vi "Modbus PreCondition.vi"(9 "Blower ON/OFF":bool, 10 "Absolute Time":dbl format="%#.20f", 11 "Timing in":T1 {"Absolute Time" format="%<%H:%M:%S%3u>t"; "Display Time" format="%#.20f"; "Test Time Ref" format="%#.20f"; "Precondition Time Ref" format="%#.20f"; "First Call Time Ref" format="%#.20f"}) -> (3 "Timing Out":T1 {"Absolute Time" format="%<%H:%M:%S%3u>t"; "Display Time" format="%#.20f"; "Test Time Ref" format="%#.20f"; "Precondition Time Ref" format="%#.20f"; "First Call Time Ref" format="%#.20f"})   [LabVIEW 2023, in "Modbus.lvlib"]
uses:
  Modbus.lvlib
  Modbus Timing.ctl
  <vilib>/Utility/miscctls.llb/LVDateTimeRec.ctl
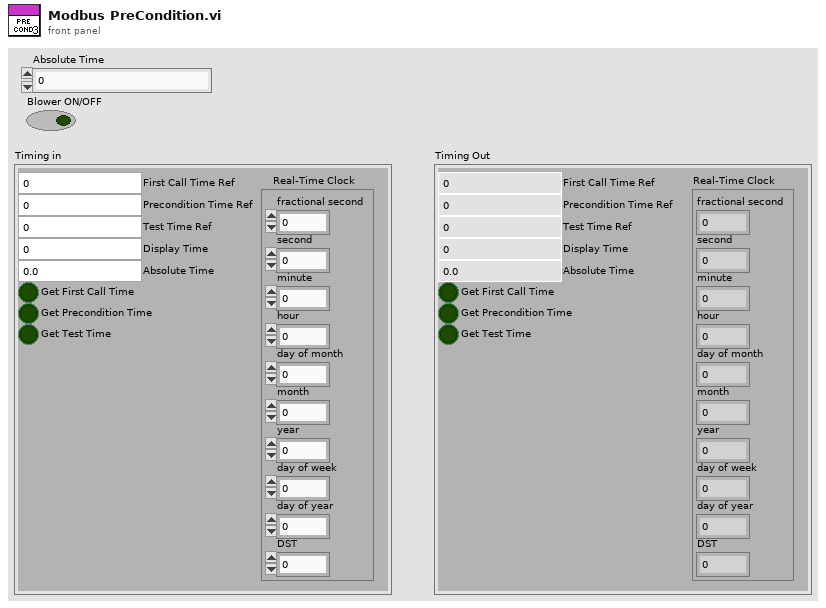
[diagram p1: front panel]
types:
  T1 = typedef "Modbus Timing.ctl" = cluster{"First Call Time Ref":dbl, "Precondition Time Ref":dbl, "Test Time Ref":dbl, "Get First Call Time":bool, "Get Precondition Time":bool, "Get Test Time":bool, "Display Time":dbl, "Real-Time Clock":T2, "Absolute Time":dbl}
  T2 = typedef "LVDateTimeRec.ctl" = cluster{"fractional second":dbl, "second":i32, "minute":i32, "hour":i32, "day of month":i32, "month":i32, "year":i32, "day of week":i32, "day of year":i32, "DST":i32}
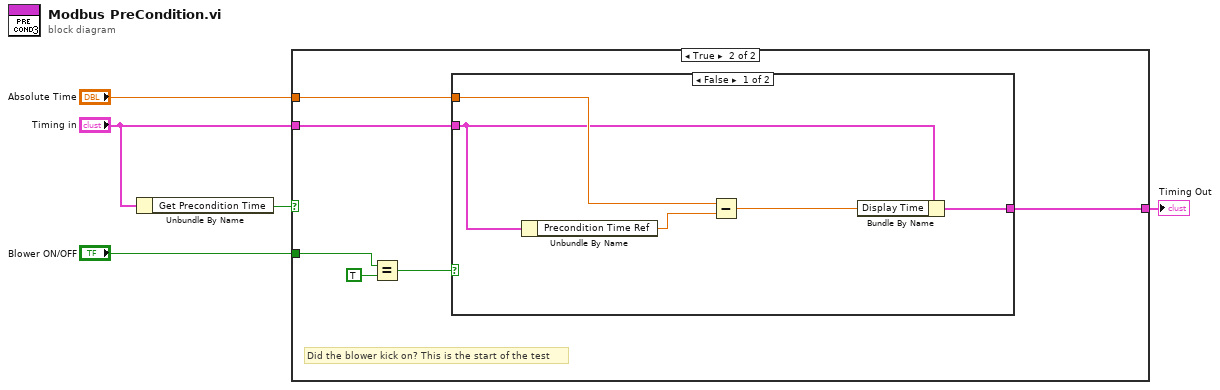
[diagram p0: block diagram]
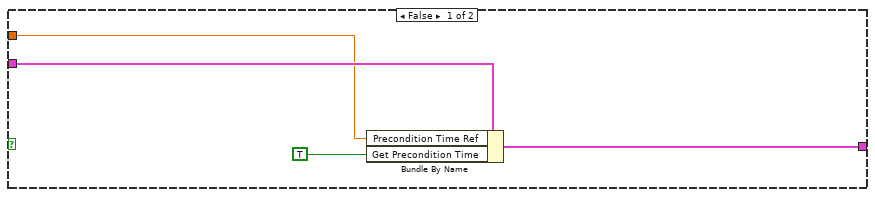
[diagram p2: hidden frame]
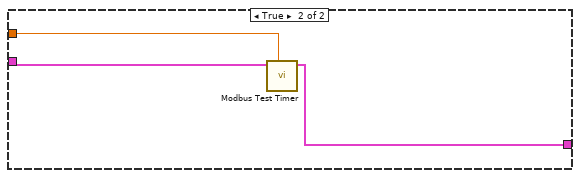
[diagram p3: hidden frame]
diagram:
  n1 = Unbundle By Name("Timing in") -> ("Get Precondition Time"=w4:bool)
  n2 = case shown="True" w4 {
    tunnel: "Timing in" -> [w9 w13]
    tunnel: [w8 w14] -> w1
    tunnel: "Absolute Time" -> [w7 w15]
    tunnel: "Blower ON/OFF" -> [_ w10]
    frame False {
      n3 = Bundle By Name(cluster=w9, "Precondition Time Ref"=w7, "Get Precondition Time"=TRUE) -> (w8:T1)
    }
    frame True {
      # "Did the blower kick on? This is the start of the test"
      n4 = Equal?(x=w10, y=TRUE) -> (x = y?=w11:bool)
      n5 = case shown="False" w11 {
        tunnel: w15 -> [w20 w21]
        tunnel: [w18 w23] -> w14
        tunnel: w13 -> [w17 w22]
        frame False {
          n6 = Unbundle By Name(w17) -> ("Precondition Time Ref"=w19:dbl)
          n7 = Subtract(x=w20, y=w19) -> (x-y=w16:dbl)
          n8 = Bundle By Name(cluster=w17, "Display Time"=w16) -> (w18:T1)
        }
        frame True {
          n9 = call "Modbus Test Timer.vi"("Absolute Time"=w21, "Timing in"=w22) -> ("Timing Out"=w23:T1)  [unwired: 9 in]
        }
      }
    }
  }
  "Timing Out" <- w1
